vi "setAngleDir_07.vi"(0 "Angle (deg)":dbl=20.0 format="%.1f", 1 "dAngle (deg)":dbl=10.0 format="%.1f", 2 "time to wait (s)":dbl=2.0, 3 "Move to ref angle first":bool, 4 "IO error in":errorcluster) -> (5 "IO error out":errorcluster)   [LabVIEW 2011]
uses:
  <vilib>/Platform/TimedLoop/XDataNode/timing_clust.ctl
  <vilib>/Platform/TimedLoop/XDataNode/nitl_modes.ctl
  <vilib>/Platform/TimedLoop/XDataNode/wakeup.ctl
  <vilib>/Platform/TimedLoop/XDataNode/XDataNode.xnode
  <vilib>/Platform/TimedLoop/XDataNode/XDNodeRunTimeDep.lvlib
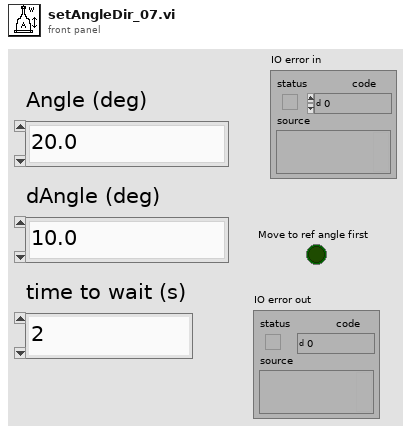
[diagram p1: front panel]
types:
  T1 = typedef "XDNodeRunTimeDep.lvlib/timing_clust.ctl" = cluster{"Expected End [f-1]":u64, "Actual End [f-1]":u64, "Finished Late? [f-1]":bool, "Expected End [i-1]":u64, "Actual End [i-1]":u64, "Finished Late? [i-1]":bool, "Expected Start [i]":u64, "Actual Start [i]":u64, "Expected Start [f]":u64, "Actual Start [f]":u64, "Source Name":string, "Structure Name":string, "Period":i64, "Deadline":i64, "Offset":i64, "Start":i64, "Priority":i32, "Timeout":i32, "Mode":T2, "Wakeup Reason":T3, "Error":errorcluster, "Source Type":string, "Secondary Source Type":string, "Global End Time":u64, "Global Start Time":u64, "Frame Duration":u64, "Iteration Duration":u64, "Assigned CPU":i32, "I/O Scan Engine Mode":u32}
  T2 = typedef "XDNodeRunTimeDep.lvlib/nitl_modes.ctl" = enum32{"No Change", "Process missed periods, maintain original phase", "Discard missed periods, maintain original phase", "Process missed periods, ignore original phase", "Discard missed periods, ignore original phase"}
  T3 = typedef "XDNodeRunTimeDep.lvlib/wakeup.ctl" = enum32{"Normal", "Aborted", "Asynchronous wakeup", "Timing source error", "Timed loop error", "Timeout"}
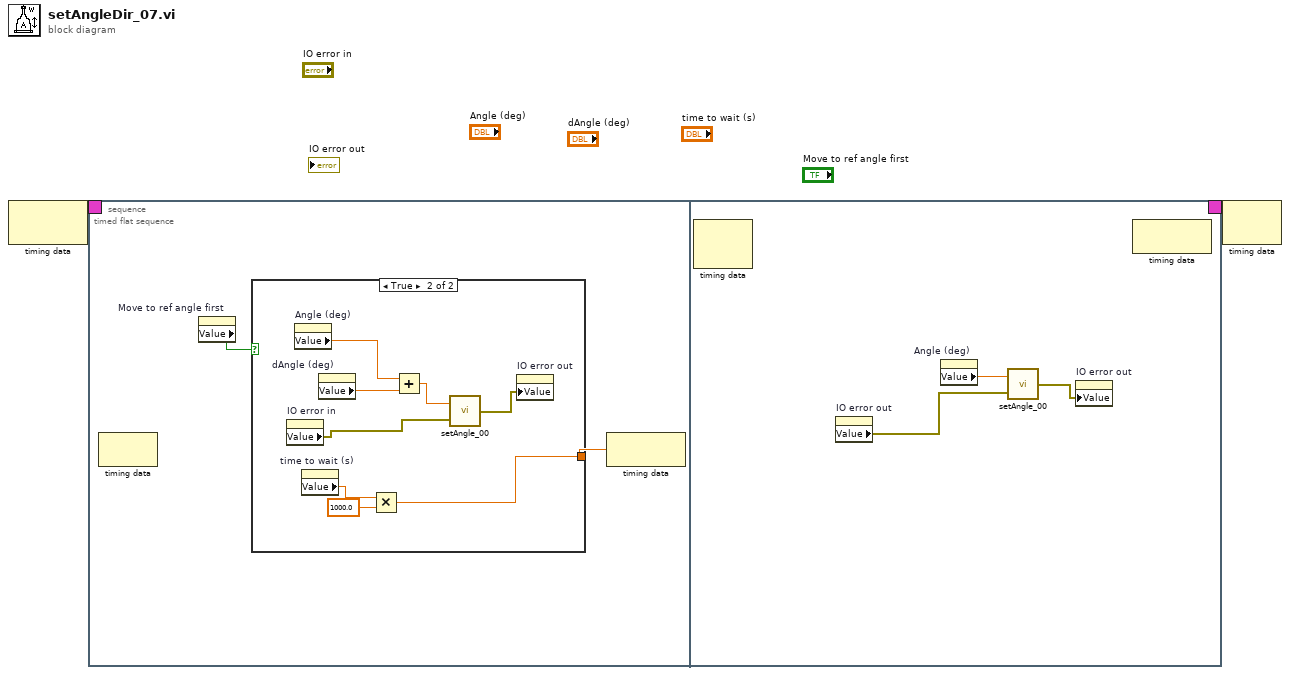
[diagram p0: block diagram]
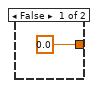
[diagram p2: hidden frame]
diagram:
  n1 = node-c288() -> (w2:T1)  [unwired: 1 in]
  n2 = timed-sequence {
    timing: w2 -> [_]
    timing-out: [_] -> w1
    n3 = timed-flat-sequence {
      frame #0 {
        n4 = node-c288() -> ()  [unwired: 1 in, 1 out]
        n5 = property on="Move to ref angle first" class="Bool (strict)"() -> ("Value"=w4:bool)  [unwired: 2 in, 2 out]
        n6 = case shown="True" w4 {
          tunnel: [0.0 ("Value") w8] -> w3
          frame False {
          }
          frame True {
            n7 = property on="IO error in" class="Clust (strict)"() -> ("Value"=w6:errorcluster)  [unwired: 2 in, 2 out]
            n8 = property on="Angle (deg)" class="DigNum (strict)"() -> ("Value"=w12:dbl)  [unwired: 2 in, 2 out]
            n9 = property on="time to wait (s)" class="DigNum (strict)"() -> ("Value"=w10:dbl)  [unwired: 2 in, 2 out]
            n10 = property on="dAngle (deg)" class="DigNum (strict)"() -> ("Value"=w13:dbl)  [unwired: 2 in, 2 out]
            n11 = Multiply(x=w10, y=1000.0) -> (x*y=w8:dbl)
            n12 = Add(x=w12, y=w13) -> (x+y=w11:dbl)
            n13 = call "setAngle_00.vi"("error in (no error)"=w6, "Angle (deg)"=w11) -> ("error out"=w7:errorcluster)
            n14 = property on="IO error out" class="Clust (strict)"("Value"=w7) -> ()  [unwired: 2 in, 2 out]
          }
        }
        n15 = node-c288(w3) -> ()  [unwired: 1 out]
      }
      frame #1 {
        n16 = node-c288() -> ()  [unwired: 1 in, 2 out]
        n17 = property on="IO error out" class="Clust (strict)"() -> ("Value"=w19:errorcluster)  [unwired: 2 in, 2 out]
        n18 = property on="Angle (deg)" class="DigNum (strict)"() -> ("Value"=w18:dbl)  [unwired: 2 in, 2 out]
        n19 = call "setAngle_00.vi"("error in (no error)"=w19, "Angle (deg)"=w18) -> ("error out"=w20:errorcluster)
        n20 = property on="IO error out" class="Clust (strict)"("Value"=w20) -> ()  [unwired: 2 in, 2 out]
        n21 = node-c288() -> ()  [unwired: 1 in, 1 out]
      }
    }
  }
  n22 = node-c288(w1) -> ()  [unwired: 1 out]
